vi "niFpgaFFTStreamingStages_32.vi"(0 "reset":bool, 1 "mult output type":fxp<+/-,18,2> format="%#.17g", 2 "bf bullet type":fxp<+,7,7>, 5 "bf data in":T1 {"x_r" format="%.16g"; "x_i" format="%.16g"; "y_r" format="%.16g"; "y_i" format="%.16g"}, 7 "stage switch in":bool, 9 "twiddle index in":fxp<+,6,6>, 11 "bf data type":T1 {"x_r" format="%.16g"; "x_i" format="%.16g"; "y_r" format="%.16g"; "y_i" format="%.16g"}) -> (6 "bf data out":T1 {"x_r" format="%.16g"; "x_i" format="%.16g"; "y_r" format="%.16g"; "y_i" format="%.16g"}, 8 "stage switch out":bool)   [LabVIEW 2017]
uses:
  <vilib>/rvi/Analysis/measure/FFT/supportingXNodes/BFGroup/templates/niFPGA BFGroup Input Buffer 32 U32.vi
  <vilib>/rvi/Analysis/measure/FFT/supportingXNodes/BFGroup/templates/niFPGA BFGroup Twiddle Table 16 U32.vi
  <vilib>/rvi/Analysis/measure/FFT/supportingXNodes/BFGroup/templates/niFPGA BFGroup Twiddle Table 4 U32.vi
  <vilib>/rvi/Analysis/measure/FFT/supportingXNodes/BFGroup/XNode/niFpgaFFTBFGroup.xnode
  <vilib>/rvi/FXPMathLib/basic elements/FxpDiscreteDelay/XNode/nifxpmath_DiscreteDelay.xnode
  <vilib>/rvi/Analysis/measure/FFT/supportingXNodes/permutation/XNode/niFpgaFFTPermutation.xnode
  <vilib>/rvi/Analysis/measure/FFT/supportingXNodes/butterfly/XNode/niFpgaFFTDIFButterfly.xnode
  <vilib>/rvi/FXPMathLib/FxpMul/XNode/nifxpmath_Multiplier.xnode
  <vilib>/rvi/FXPMathLib/sim/FxpSim.dll
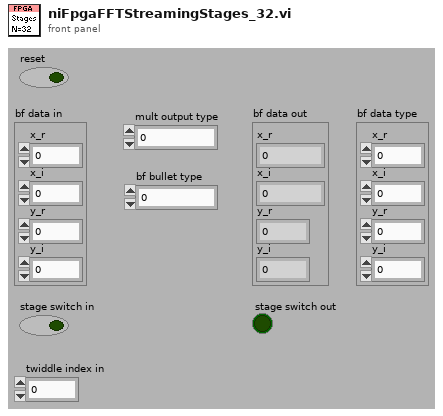
[diagram p1: front panel]
types:
  T1 = cluster{"x_r":fxp<+/-,16,1>, "x_i ":fxp<+/-,16,1>, "y_r ":fxp<+/-,16,1>, "y_i ":fxp<+/-,16,1>}
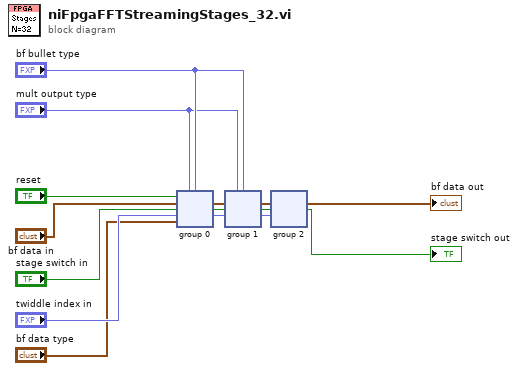
[diagram p0: block diagram]
diagram:
  n1 = xnode "group 0"("mult output type"="mult output type", "bf data in"="bf data in", "stage switch in"="stage switch in", "tf index in"="twiddle index in", "reset"="reset", "bf bullet type"="bf bullet type", "bf data type"="bf data type") -> ("stage switch out"=w11:bool, "bf data out"=w13:T1, "tf index out"=w12:fxp<+,4,4>)
  n2 = xnode "group 1"("mult output type"="mult output type", "bf data in"=w13, "stage switch in"=w11, "tf index in"=w12, "bf bullet type"="bf bullet type") -> ("stage switch out"=w9:bool, "bf data out"=w10:T1, "tf index out"=w8:fxp<+,4,4>)
  n3 = xnode "group 2"("bf data in"=w10, "stage switch in"=w9, "tf index in"=w8) -> ("stage switch out"=→"stage switch out":bool, "bf data out"=→"bf data out":T1)
